vi "Z Aux Direct Get In.vi"(8 "error in (no error)":errorcluster caption="错误输入（无错误）", 9 "piValue":u32, 10 "ionum":i32, 11 "handle":u32) -> (0 "error out":errorcluster caption="错误输出", 1 "piValue out":u32, 2 "function return":i32, 3 "handle out":u32)   [LabVIEW 2015, in "zauxdll.lvlib"]
doc: "int32 __stdcall ZAux_Direct_GetIn(ZMC_HANDLE handle, int ionum , uint32 *piValue);"
uses:
  zauxdll.lvlib
  zauxdll.dll
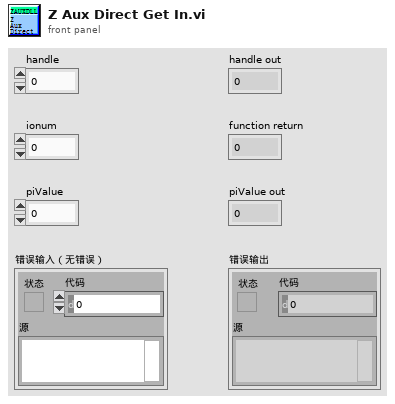
[diagram p1: front panel]
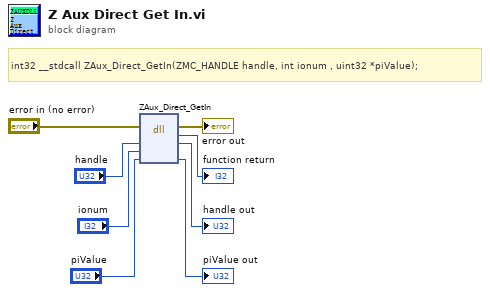
[diagram p0: block diagram]
diagram:
  # "int32 __stdcall ZAux_Direct_GetIn(ZMC_HANDLE handle, int ionum , uint32 *piValue);"
  n1 = dll-call lib="C:/Users/VIC/Desktop/GOGORO_Oringnal - Panasonic/system/LLB/zmotion/zaux/zauxdll.*" fn="ZAux_Direct_GetIn"(error in="error in (no error)", "handle"="handle", "ionum"="ionum", "piValue"="piValue") -> (error out=→"error out":errorcluster, →"function return":i32, "handle"=→"handle out":u32, "piValue"=→"piValue out":u32)  [unwired: 3 in, 1 out]
